vi "BBB Main.vi"() -> ()   [LabVIEW 2019]
uses:
  <vilib>/MakerHub/LINX/Public/Peripherals/Digital/Digital Write 1 Chan.vi
  <vilib>/MakerHub/LINX/Public/Peripherals/Digital/Digital Write N Chans.vi
  <vilib>/MakerHub/LINX/Private/Local IO/LinxDigitalWrite.vi
  <vilib>/MakerHub/LINX/Public/Utilities/Check Channel.vi
  <vilib>/MakerHub/LINX/Public/Utilities/Open Local.vi
  <vilib>/MakerHub/LINX/Private/Utilties/Generate Error.vi
  <vilib>/MakerHub/LINX/LMH-LINX.lvlib
panel:
  in  "Click Me!":bool
  in  "DO Channel":u8=7
  in  "Stop Button":bool
  # "BeagleBone Black Blink!\n\nUse this VI to blink and LED connected to the specified digital output channel.\n1. Connect an LED to pin 7 and ground as shown in the image below.\n2. Click the round LED control below to blink the LED.\n\nFor more details on the BeagleBone Black LINX channels visit labviewmakerhub.com/linx/beaglebone-black\nVisit labviewmakerhub.com/forums/linx to get help and share your projects."
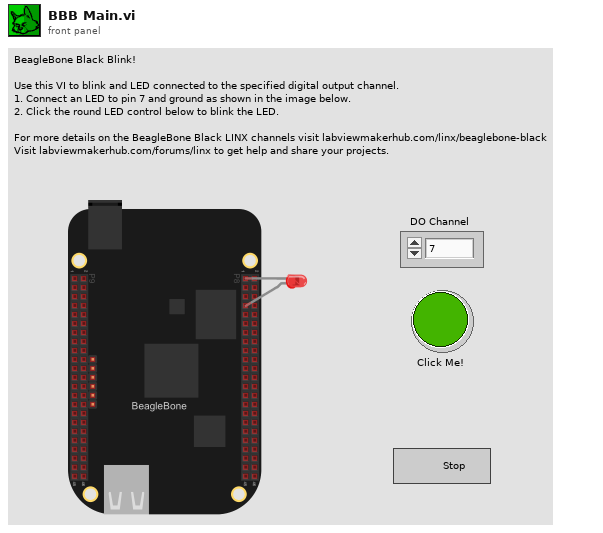
[diagram p1: front panel]
types:
  T1 = typedef "LMH-LINX.lvlib/LINX Ref.ctl" = cluster{"IO":T2, "Interface":T3, "LINX Device Config":T4}
  T2 = typedef "LMH-LINX.lvlib/Platform.ctl" = enum16{"Remote", "Local"}
  T3 = typedef "LMH-LINX.lvlib/Interface.ctl" = enum16{"Serial", "TCP"}
  T4 = typedef "LMH-LINX.lvlib/Device.lvlib/LINX Device Config.ctl" = cluster{"Interface":T3, "COM Port":refnum<visa-resource-name>, "TCP Configuration":T5, "Device Family":u8, "Device ID":u8, "Device Name":string, "TCP Ref":refnum<k5>, "Channels":T6}
  T5 = typedef "LMH-LINX.lvlib/Device.lvlib/TCP Config.ctl" = cluster{"IP Address":string, "Port":u16}
  T6 = typedef "LMH-LINX.lvlib/Channels.ctl" = cluster{"DI":u8[], "DO":u8[], "AI":u8[], "AO":u8[], "PWM":u8[], "QE":u8[], "UART":u8[], "I2C 2":u8[], "SPI":u8[], "CAN":u8[], "Servo":u8[], "AI Ref (V)":dbl, "AI Resolution (Bits)":u8, "AO Ref (V)":dbl, "AO Resolution (Bits)":u8}
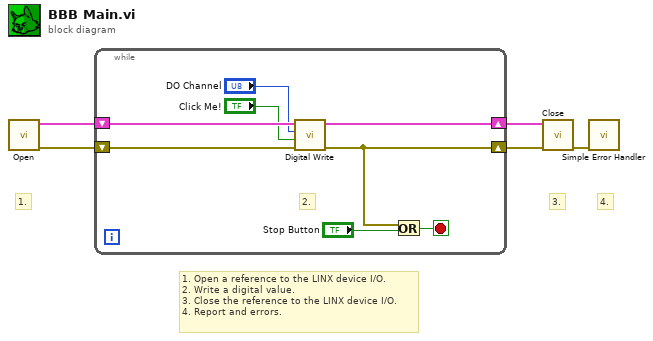
[diagram p0: block diagram]
diagram:
  # "4."
  # "3."
  # "1."
  # "1. Open a reference to the LINX device I/O.\n2. Write a digital value.\n3. Close the reference to the LINX device I/O.\n4. Report and errors."
  n1 = call-poly <vilib>:"Open.vi"() -> ("Error Out"=w2:errorcluster, "LINX Resource"=w5:T1)  [unwired: 9 in, 1 out]
  n2 = while {
    shift-right: [w12] -> w4
    shift-left: w5 -> [w13]
    shift-right: [w9] -> w3
    shift-left: w2 -> [w11]
    stop <- w10 stop-if-true
    # "2."
    n3 = call-poly <vilib>:"Digital Write.vi"("Error In"=w11, "Output Value"="Click Me!", "DO Channel"="DO Channel", "LINX Resource"=w13) -> ("Error Out"=w9:errorcluster, "LINX Resource"=w12:T1)  [unwired: 6 in]
    n4 = Or(x=w9, y="Stop Button") -> (x .or. y?=w10:bool)
  }
  n5 = call <vilib>:"Close.vi"("Error In"=w3, "LINX Resource"=w4) -> ("Error Out"=w1:errorcluster)  [unwired: 9 in]
  n6 = call <vilib>:"Simple Error Handler.vi"("error in (no error)"=w1) -> ()  [unwired: 4 in, 5 out]
